vi "makeORTCurve.vi"(10 "cantileverParams":T1={"samplingRate"=300.0, "cantileverFreq"=500000.0, "qFactor"=10.0} {"cantileverFreq" format="%#_6p"; "samplingRate" format="%#_6p"}, 11 "curveParams":T2={"amplitude"=2000.0, "peakHeight"=200.0, "cycleLength"=0, "snapIn"=10.0, "adhesion"=300.0, "peakShift"=200, "noiseAmplitude"=10.0, "asymmetry"=0.5}) -> (3 "ortCurve":dbl[](array[numeric]))   [LabVIEW 2016]
uses:
  <vilib>/addons/Control Design/_Model Construction/Model Creation.llb/Model Creation SubVI/cd_Create State Space Model.vi
  <vilib>/addons/Control Design/_Time Response Analysis/Time Response.llb/Time Response subVI/cd_Linear Simulation (State-Space).vi
  <vilib>/Analysis/NI_AALBase.lvlib
  <vilib>/addons/Control Design/_Time Response Analysis/NI_CD_Time Response.lvlib
  <vilib>/addons/Control Design/_Model Construction/NI_LinSys_Model Creation.lvlib
panel:
  out "Waveform Graph":dbl[](graph)
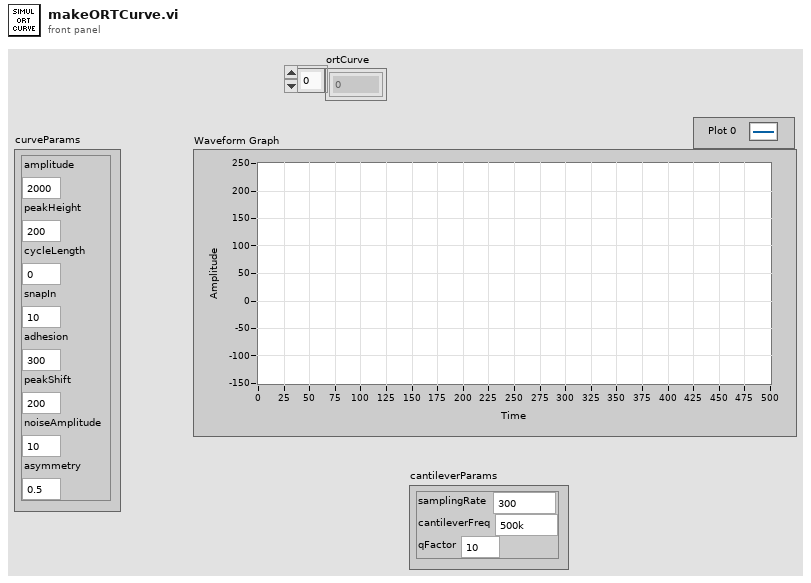
[diagram p1: front panel]
types:
  T1 = cluster{"samplingRate":dbl, "cantileverFreq":dbl, "qFactor":dbl}
  T2 = cluster{"amplitude":dbl, "peakHeight":dbl, "cycleLength":u16, "snapIn":dbl, "adhesion":dbl, "peakShift":u16, "noiseAmplitude":dbl, "asymmetry":dbl}
  T3 = typedef "NI_LinSys_Model Typedefs.lvlib/CD State Space Model (MIMO).ctl" = cluster{"properties":T4, "A":dbl[][], "B":dbl[][], "C":dbl[][], "D":dbl[][], "StateNames":string[], "Transport Delay":dbl[][]}
  T4 = typedef "NI_LinSys_Model Typedefs.lvlib/CD General Elements.ctl" = cluster{"Model name":string, "Input names":string[], "Output names":string[], "Input Delays":dbl[], "Output Delays":dbl[], "Sampling Time":dbl, "Notes":string}
  T5 = typedef "NI_LinSys_Data Typedefs.lvlib/CD MIMO Time Response Data.ctl" = cluster{"Time":dbl[], "Outputs Data":dbl[][][], "States Data":dbl[][][], "plot type":T6}
  T6 = typedef "NI_LinSys_Data Typedefs.lvlib/CD Plot Types Enum.ctl" = enum16{"bode-magnitude", "bode-phase", "nichols", "nyquist", "singular values", "step", "impulse", "initial", "simulation", "nyquist with separation"}
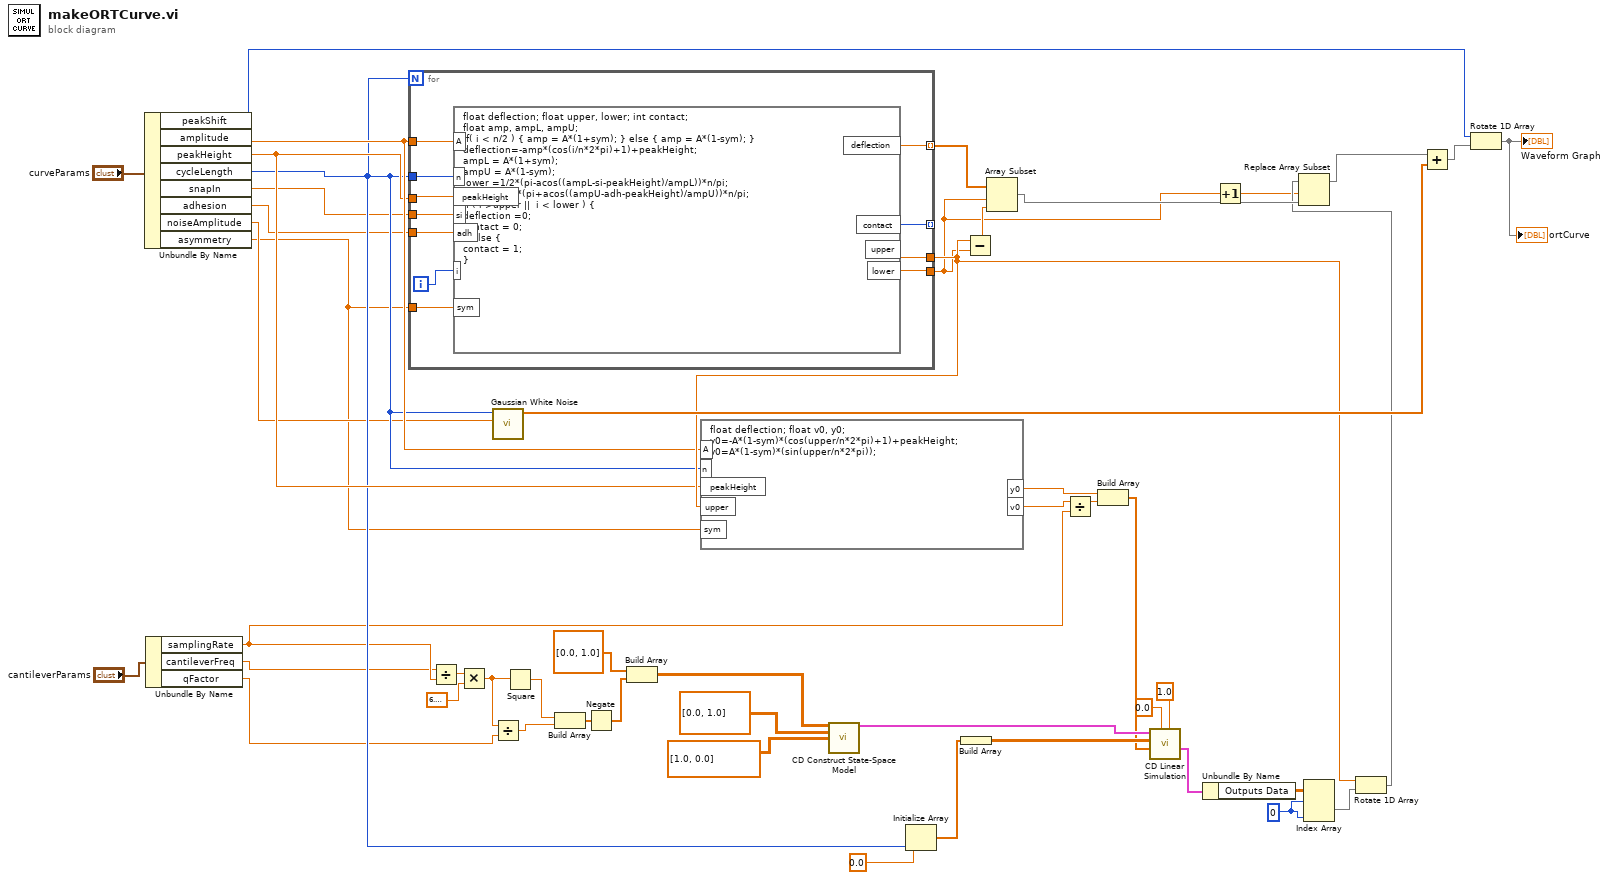
[diagram p0: block diagram]
diagram:
  w17 = 0 ("index (page)")
  n1 = Unbundle By Name("curveParams") -> ("peakShift"=w8:u16, "amplitude"=w13:dbl, "peakHeight"=w12:dbl, "cycleLength"=w11:u16, "snapIn"=w10:dbl, "adhesion"=w9:dbl, "noiseAmplitude"=w7:dbl, "asymmetry"=w2:dbl)
  n2 = Unbundle By Name("cantileverParams") -> ("samplingRate"=w5:dbl, "cantileverFreq"=w4:dbl, "qFactor"=w3:dbl)
  n3 = for {
    N: w11 -> [_]
    tunnel: w11 -> [w60]
    tunnel: w13 -> [w59]
    tunnel: [w57] -> w22 mode=indexing
    tunnel: w12 -> [w56]
    tunnel: w10 -> [w55]
    tunnel: w9 -> [w54]
    tunnel: [w53] -> _ mode=indexing
    tunnel: [w52] -> w19
    tunnel: [w51] -> w16
    tunnel: w2 -> [w50]
    i -> [w58]
    n4 = formula code="float deflection; float upper, lower; int contact; \nfloat amp, ampL, ampU;\nif( i < n/2 ) { amp = A*(1+sym); } else { amp = A*(1-sym); }\ndeflection=-amp*(cos(i/n*2*pi)+1)+peakHeight;\nampL = A*(1+sym);\nampU = A*(1-sym);\nlower =1/2*(pi-acos((ampL-si-peakHeight)/ampL))*n/pi;\nupper =1/2*(pi+acos((ampU-adh-peakHeight)/ampU))*n/pi;\nif ( i >upper ||  i < lower ) {\ndeflection =0;\ncontact = 0;\n} else {\ncontact = 1;\n}"("A"=w59, "n"=w60, "i"=w58, "peakHeight"=w56, "si"=w55, "adh"=w54, "sym"=w50) -> ("deflection"=w57:dbl, "contact"=w53:i32, "upper"=w52:dbl, "lower"=w51:dbl)
  }
  n5 = Divide(x=w4, y=w5) -> (x/y=w45:dbl)
  n6 = Multiply(x=w45, y=6.283185307179586) -> (x*y=w35:dbl)
  n7 = call <vilib>:"Gaussian White Noise.vi"("standard deviation"=w7, "samples"=w11) -> ("Gaussian noise pattern"=w48:dbl[])  [unwired: 8 in, 1 out]
  n8 = Divide(x=w35, y=w3) -> (x/y=w34:dbl)
  n9 = Square(x=w35) -> (x^2=w46:dbl)
  n10 = Build Array(w46, w34) -> (w33:dbl[])
  n11 = Negate(x=w33) -> (-x=w27:dbl[])
  n12 = Build Array(dbl[] [0.0, 1.0] ("appended array"), w27) -> (w31:dbl[][])
  n13 = formula code="float deflection; float v0, y0;\ny0=-A*(1-sym)*(cos(upper/n*2*pi)+1)+peakHeight;\nv0=A*(1-sym)*(sin(upper/n*2*pi));"("A"=w13, "n"=w11, "peakHeight"=w12, "upper"=w19, "sym"=w2) -> ("y0"=w30:dbl, "v0"=w29:dbl)
  n14 = call-poly <vilib>:"CD Construct State-Space Model.vi"("A"=w31, "B"=dbl[][] [[0.0], [1.0]], "C"=dbl[][] [[1.0, 0.0]]) -> ("State-Space Model"=w38:T3)  [unwired: 11 in, 1 out]
  n15 = Initialize Array(0.0 ("element"), w11) -> (w40:dbl[])
  n16 = Build Array(w40) -> (w39:dbl[][])
  n17 = Subtract(x=w19, y=w16) -> (x-y=w21:dbl)
  n18 = Array Subset(array=w22, index=w16, length=w21) -> (w20:dbl[])
  n19 = Divide(x=w29, y=w5) -> (x/y=w26:dbl)
  n20 = Build Array(w30, w26) -> (w28:dbl[])
  n21 = call-poly <vilib>:"CD Linear Simulation.vi"("Delta t"=1.0, "Initial Time"=0.0 ("Initial time"), "Initial Conditions"=w28, "Inputs"=w39, "State-Space Model"=w38) -> ("Simulation Data"=w25:T5)  [unwired: 3 in, 3 out]
  n22 = Unbundle By Name(w25) -> ("Outputs Data"=w24:dbl[][][])
  n23 = Increment(x=w16) -> (x+1=w1:dbl)
  n24 = Index Array(array=w24, index (dim 0)=w17, index (dim 2)=w17) -> (element=w23:dbl[])  [unwired: 1 in]
  n25 = Rotate 1D Array(1:w23, 2:w19) -> (0:w15:dbl[])
  n26 = Replace Array Subset(array=w15, new element=w20, index=w1) -> (w18:dbl[])
  n27 = Add(x=w18, y=w48) -> (x+y=w47:dbl[])
  n28 = Rotate 1D Array(1:w47, 2:w8) -> (0:→"Waveform Graph" →"ortCurve":dbl[])
